vi "备用系数读取.vi"(8 "error in (no error)":errorcluster caption="错误输入（无错误）", 9 "量程":enum16{"低量程", "高量程"}(ring), 10 "测量模式":T1(ring), 11 "测量参数":u16(ring) items=["COD"=22, "氨氮"=3, "总氮"=2, "总磷"=1]) -> (0 "error out":errorcluster caption="错误输出", 3 "备用系数":cluster{"上限":dbl, "下限":dbl, "范围":dbl})   [LabVIEW 2016, in "斯坦道总磷.lvlib"]
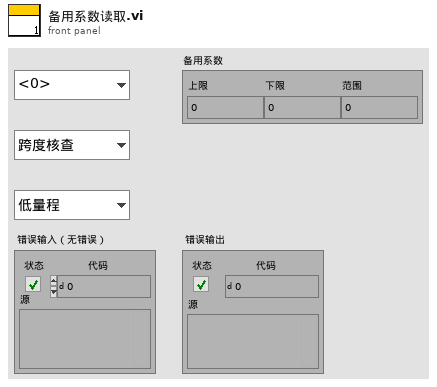
[diagram p1: front panel]
types:
  T1 = enum16{"跨度核查", "水样测量", "零点核查", "标样核查", "加标回收", "快捷测试", "空白校准", "标样校准"}
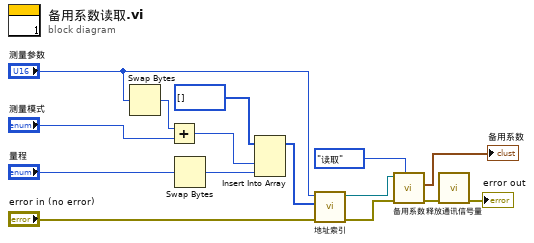
[diagram p0: block diagram]
diagram:
  n1 = Swap Bytes(anything="测量参数") -> (byte swapped=w6:u16)
  n2 = Add(x=w6, y="测量模式") -> (x+y=w8:u16)
  n3 = Swap Bytes(anything="量程") -> (byte swapped=w5:u16)
  n4 = Insert Into Array(array=u16[] [] ("数组"), new element #1=w8, new element #2=w5) -> (w1:u16[])  [unwired: 1 in]
  n5 = call "地址索引.vi"("error in (no error)"="error in (no error)", "values"=w1, "测量参数"="测量参数") -> ("error out"=w14:errorcluster, "MB session out"=w15:refnum<class "MB_Master.lvclass">)  [unwired: 7 in]
  n6 = call "备用系数.vi"("功能"=enum16{"读取", "写入"}."读取", "error in (no error)"=w14, "MB session in"=w15) -> ("error out"=w9:errorcluster, "备用系数读取"=→"备用系数":cluster{"上限":dbl, "下限":dbl, "范围":dbl})  [unwired: 6 in, 1 out]
  n7 = call "释放通讯信号量.vi"("error in (no error)"=w9) -> ("error out"=→"error out":errorcluster)  [unwired: 10 in]
